vi "CoMP-S TDMS Cbk Array Convertor.vi"(6 "Comments":string, 7 "date/time string":string, 8 "Arg 3":path, 9 "Arg 2":sgl, 10 "Arg 1":sgl, 11 "Data Type":T1(ring)) -> (1 "TDMS Data Output":string[][](array[string]), 2 "TDMS Channel Name":string[](array[string]))   [LabVIEW 2014]
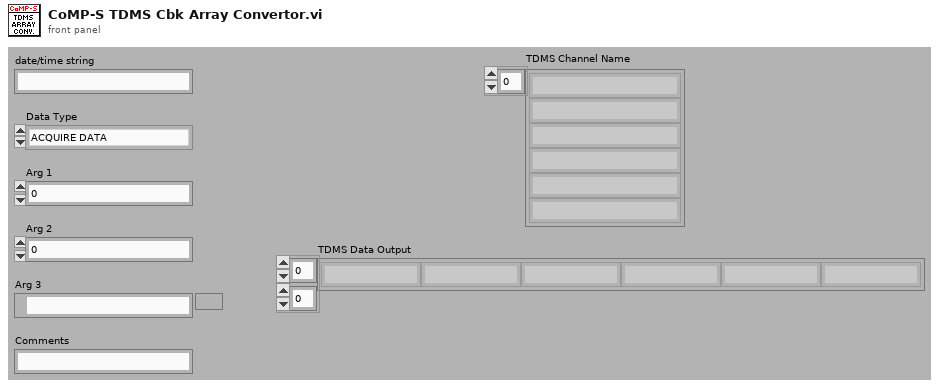
[diagram p1: front panel]
types:
  T1 = enum32{"ACQUIRE DATA", "SET DIFFUSER", "CAL-FW", "WAVELENGTH-FW", "INSTR. ROTATION", "SET FOCUS", "DATATYPE", "SET EXPOSURE", "CBK COMMENTS"}
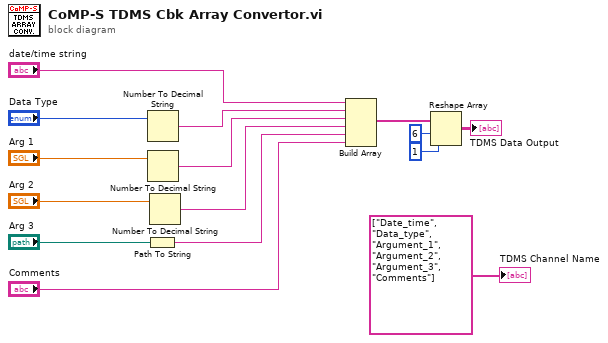
[diagram p0: block diagram]
diagram:
  n1 = Path To String(path="Arg 3") -> (string=w14:string)
  n2 = Number To Decimal String(number="Data Type") -> (decimal integer string=w11:string)  [unwired: 1 in]
  n3 = Number To Decimal String(number="Arg 1") -> (decimal integer string=w12:string)  [unwired: 1 in]
  n4 = Number To Decimal String(number="Arg 2") -> (decimal integer string=w13:string)  [unwired: 1 in]
  n5 = Build Array("date/time string", w11, w12, w13, w14, "Comments") -> (w5:string[])
  n6 = Reshape Array(w5, 6 ("dimension size"), 1 ("dimension size")) -> (→"TDMS Data Output":string[][])
  "TDMS Channel Name" <- string[] ["Date_time", "Data_type", "Argument_1", "Argument_2", "Argument_3", "Comments"] ("Channel Name")
